vi "UpdateVariablesTCLastAcquire.vi"(8 "error in (no error)":errorcluster, 9 "SignificantDigits (8)":u32=8, 10 "Format (SI notation)":T1(ring)=enum."SI notation", 11 "VMUI in":refnum<class "VMUI.lvclass">) -> (0 "error out":errorcluster, 3 "VMUI out":refnum<class "VMUI.lvclass">)   [LabVIEW 2013, in "VMUI.lvclass"]
uses:
  VMUI.lvclass
  VariableManager/VariableManager.lvclass
  VariableValue/VariableValue.lvclass
  API/VariableManagerAPI.lvlib
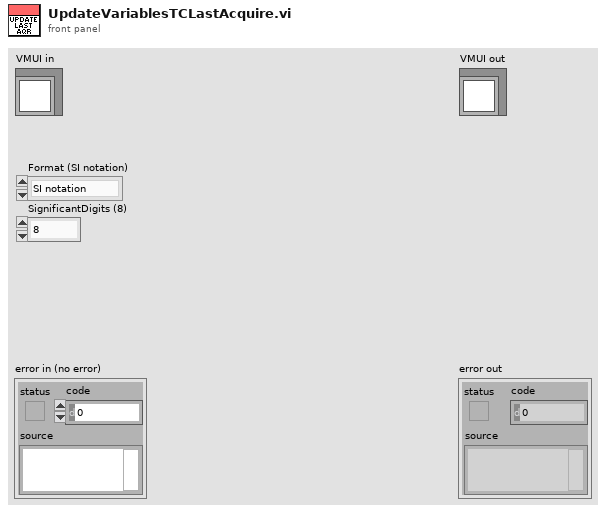
[diagram p1: front panel]
types:
  T1 = enum16{"Floating point", "Scientific SI", "Automatic SI", "SI notation"}
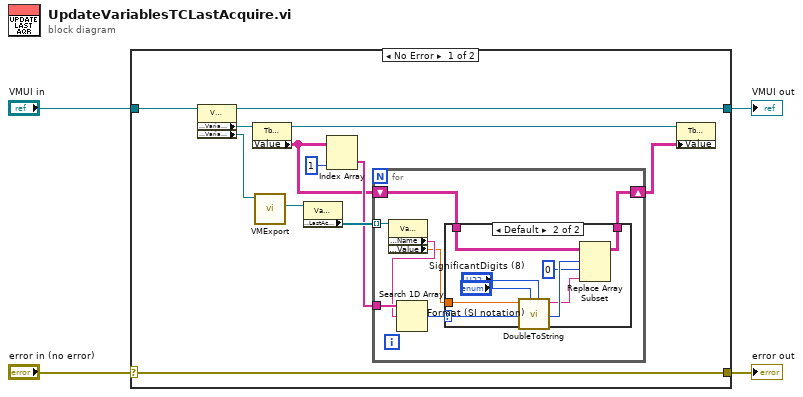
[diagram p0: block diagram]
diagram:
  n1 = case shown="No Error" "error in (no error)" {
    selector: "error in (no error)" -> [w16 w34]
    tunnel: [w16 w34] -> w3
    tunnel: [w14 w33] -> w1
    tunnel: "VMUI in" -> [w15 w33]
    frame No Error {
      n2 = property class="VMUI.lvclass"(reference=w15) -> (reference out=w14:refnum<class "VMUI.lvclass">, "Accessors:VariablesTCRef"=w13:refnum<vi>, "Accessors:VariableManagerRef"=w6:refnum<vi>)  [unwired: 1 in, 1 out]
      n3 = property class="Tbl (strict)"(reference=w13) -> (reference out=w8:refnum<vi>, "Value"=w9:string[][])  [unwired: 1 in, 1 out]
      n4 = call "VMExport.vi"("VariableManagerRef in"=w6) -> ("VariableManagerExportCopy"=w5:refnum<class "VariableManager.lvclass">)  [unwired: 8 in, 2 out]
      n5 = property class="VariableManager.lvclass"(reference=w5) -> ("Accessors:LastAcquireValues"=w12:refnum<class "VariableValue.lvclass">[])  [unwired: 1 in, 2 out]
      n6 = Index Array(array=w9, index (col)=1 ("disabled index (col)")) -> (element=w10:string[])  [unwired: 1 in]
      n7 = for {
        tunnel: w12 -> [w23] mode=indexing
        tunnel: w10 -> [w22]
        shift-right: [w17] -> w7
        shift-left: w9 -> [w18]
        n8 = property class="VariableValue.lvclass"(reference=w23) -> ("Accessors:Name"=w21:string, "Accessors:Value"=w19:dbl)  [unwired: 1 in, 2 out]
        n9 = Search 1D Array(1D array=w22, element=w21) -> (index of element=w20:i32)  [unwired: 1 in]
        n10 = case shown="Default" w20 {
          selector: w20 -> [_ w30]
          tunnel: w19 -> [_ w27]
          tunnel: w18 -> [w24 w32]
          tunnel: [w24 w31] -> w17
          frame -1 {
          }
          frame Default {
            n11 = call "DoubleToString.vi"("SignificantDigits (8)"="SignificantDigits (8)", "Format (SI notation)"="Format (SI notation)", "Double"=w27) -> ("String"=w28:string)  [unwired: 8 in]
            n12 = Replace Array Subset(array=w32, new element=w28, index (row)=w30, index (col)=0 ("disabled index (col)")) -> (w31:string[][])
          }
        }
      }
      n13 = property class="Tbl (strict)"(reference=w8, "Value"=w7) -> ()  [unwired: 1 in, 2 out]
    }
    frame Error {
    }
  }
  "error out" <- w3
  "VMUI out" <- w1
